vi "Draw Ground.vi"(7 "attitude (rad)":T1, 9 "draw options":T2={"Text Color"=16777238, "Wing Color"=16751616, "Dial Outline Color"=13816530, "Sky Color"=3381759, "Ground Color"=8213043, "Horizon Line Color"=16777225, "Outline Color"=0, "Dial Background Color"=5987163, "Draw Wings"=TRUE, "Draw Text"=TRUE, "Font Name"="Helvetica", "Angle units"=enum."Radians"}, 10 "draw area state":T4, 11 "picture in":picture) -> (3 "picture out":picture)   [LabVIEW 2017, in "NI_Robotics_Attitude Picture.lvlib"]
uses:
  <vilib>/robotics/Controls/Attitude Indicator/Attitude Picture/NI_Robotics_Attitude Picture.lvlib
  <vilib>/robotics/Controls/Attitude Indicator/Attitude Picture/Draw Area State.ctl
  <vilib>/Utility/miscctls.llb/LVBoundsTypeDef.ctl
  <vilib>/robotics/Controls/Attitude Indicator/Attitude Picture/Draw Options.ctl
  <vilib>/robotics/Controls/Utilities/Angle Units.ctl
  <vilib>/robotics/Controls/Attitude Indicator/Attitude Picture/Attitude.ctl
  <vilib>/Analysis/coordinate.llb/2D Cartesian Coordinate Rotation.vi
  <vilib>/Analysis/coordinate.llb/2D Cartesian Coordinate Rotation (Array).vi
  <vilib>/robotics/Controls/Utilities/NI_Robotics_Control Utilities.lvlib
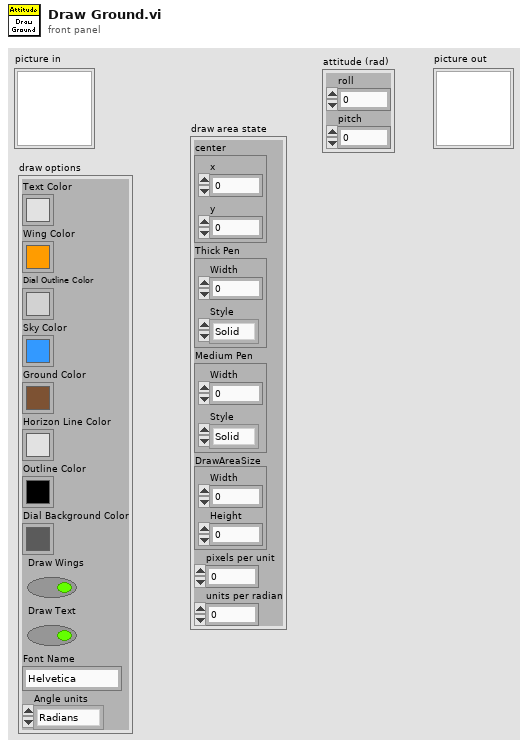
[diagram p1: front panel]
types:
  T1 = typedef "NI_Robotics_Attitude Picture.lvlib/Attitude.ctl" = cluster{"roll":dbl, "pitch":dbl}
  T2 = typedef "NI_Robotics_Attitude Picture.lvlib/Draw Options.ctl" = cluster{"Text Color":u32, "Wing Color":u32, "Dial Outline Color":u32, "Sky Color":u32, "Ground Color":u32, "Horizon Line Color":u32, "Outline Color":u32, "Dial Background Color":u32, "Draw Wings":bool, "Draw Text":bool, "Font Name":string, "Angle units":T3}
  T3 = typedef "NI_Robotics_Control Utilities.lvlib/Angle Units.ctl" = enum16{"Radians", "Degrees"}
  T4 = typedef "NI_Robotics_Attitude Picture.lvlib/Draw Area State.ctl" = cluster{"center":cluster{"x":i16, "y":i16}, "Thick Pen":cluster{"Width":u16, "Style":enum32{"Solid", "Dash", "Dot", "DashDot", "DashDotDot"}}, "Medium Pen":cluster{"Width":u16, "Style":enum32{"Solid", "Dash", "Dot", "DashDot", "DashDotDot"}}, "DrawAreaSize":T5, "pixels per unit":dbl, "units per radian":dbl}
  T5 = typedef "LVBoundsTypeDef.ctl" = cluster{"Width":u32, "Height":u32}
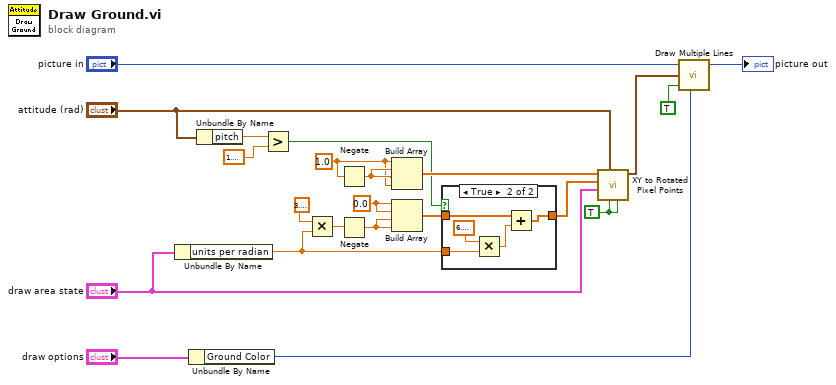
[diagram p0: block diagram]
diagram:
  w10 = TRUE ("use pitch")
  w17 = 0.0 ("element")
  w14 = 1.0 ("element")
  n1 = Unbundle By Name("draw area state") -> ("units per radian"=w1:dbl)
  n2 = Unbundle By Name("draw options") -> ("Ground Color"=w18:u32)
  n3 = Unbundle By Name("attitude (rad)") -> ("pitch"=w8:dbl)
  n4 = Greater?(x=w8, y=1.5707963267948966) -> (0:w3:bool)
  n5 = Multiply(x=3.141592653589793, y=w1) -> (x*y=w2:dbl)
  n6 = Negate(x=w14) -> (-x=w15:dbl)
  n7 = Negate(x=w2) -> (-x=w16:dbl)
  n8 = Build Array(w14, w15, w15, w14) -> (w13:dbl[])
  n9 = Build Array(w17, w17, w16, w16) -> (w6:dbl[])
  n10 = case shown="True" w3 {
    tunnel: w6 -> [w23 w28]
    tunnel: [w23 w27] -> w5
    tunnel: w1 -> [_ w25]
    frame False {
    }
    frame True {
      n11 = Multiply(x=6.283185307179586, y=w25) -> (x*y=w24:dbl)
      n12 = Add(x=w28, y=w24) -> (x+y=w27:dbl[])
    }
  }
  n13 = call <vilib>:"XY to Rotated Pixel Points.vi"("use roll"=w10, "use pitch"=w10, "attitude (rad)"="attitude (rad)", "draw area state"="draw area state", "unrotated y (units)"=w5, "unrotated x (units)"=w13) -> ("rotated pixel points"=w12:cluster{"x":i16, "y":i16}[])  [unwired: 5 in]
  n14 = call <vilib>:"Draw Multiple Lines.vi"("picture"="picture in", "line endpoints"=w12, "fill?(F)"=TRUE, "color(black)"=w18) -> ("new picture"=→"picture out":picture)  [unwired: 5 in]
